vi "RelevantVIsAndConstants.vi"() -> ()   [LabVIEW 2018]
panel:
  in  "Values List":string[](array[string])
  in  "Components List":string[](array[string])
  in  "Save Calibration Button":bool
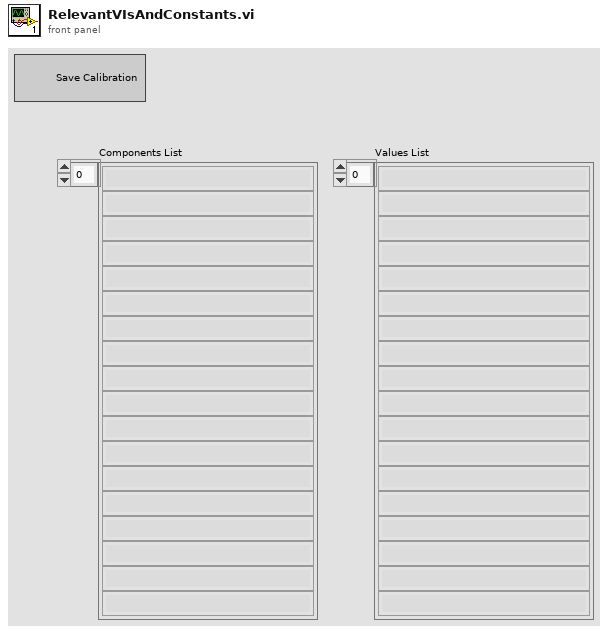
[diagram p1: front panel]
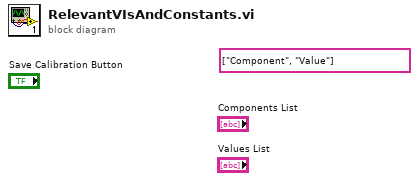
[diagram p0: block diagram]
diagram:
  (unwired) string[] ["Component", "Value"]
